vi "Timer_Check.vi"(1 "TimeLimit(ms)":u16, 4 "Timer.t0":u16) -> (16 "TimeElapsed":bool)   [LabVIEW 2018]
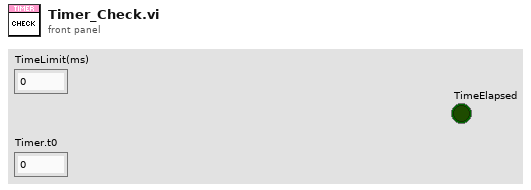
[diagram p1: front panel]
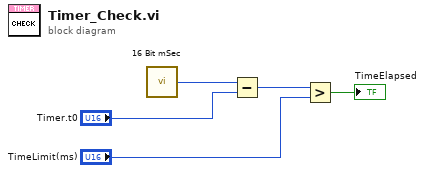
[diagram p0: block diagram]
diagram:
  n1 = call "16 Bit mSec"() -> ("Tick Count(mSec)"=w5:u16)
  n2 = Subtract(x=w5, y="Timer.t0") -> (x-y=w3:u16)
  n3 = Greater?(x=w3, y="TimeLimit(ms)") -> (0:→"TimeElapsed":bool)
